vi "CalStringToINIsketch.vi"() -> ()   [LabVIEW 2016]
uses:
  <vilib>/Utility/config.llb/NI_LVConfig.lvlib
  <vilib>/Utility/config.llb/Write Key (Boolean).vi
panel:
  in  "String":string
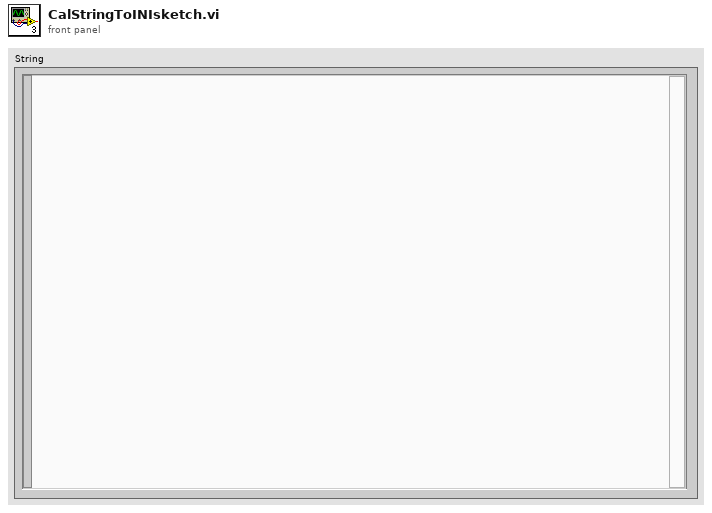
[diagram p1: front panel]
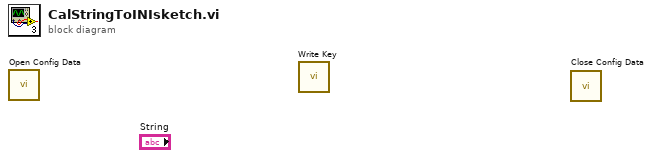
[diagram p0: block diagram]
diagram:
  n1 = call <vilib>:"Open Config Data.vi"() -> ()  [unwired: 9 in, 3 out]
  n2 = call-poly <vilib>:"Write Key.vi"() -> ()  [unwired: 9 in, 3 out]
  n3 = call <vilib>:"Close Config Data.vi"() -> ()  [unwired: 10 in, 2 out]
